vi "_PC_RTFunc_AccessLaser.vi"(7 "Function":enum16{"Init", "Write", "Read"}(ring), 8 "error in (no error)":errorcluster, 10 "Data":variant) -> (0 "error out":errorcluster, 2 "LaserSetting":T1={"Energy"=1.0, "Freq"=1.0, "Emission"=FALSE, "TriggerSource"=enum."Internal", "Time Stamp"=timestamp(0 s since 1904-01-01)})   [LabVIEW 2018]
uses:
  RT/ControlLoop/Laser/Ctl/_ctl_LaserParam.ctl
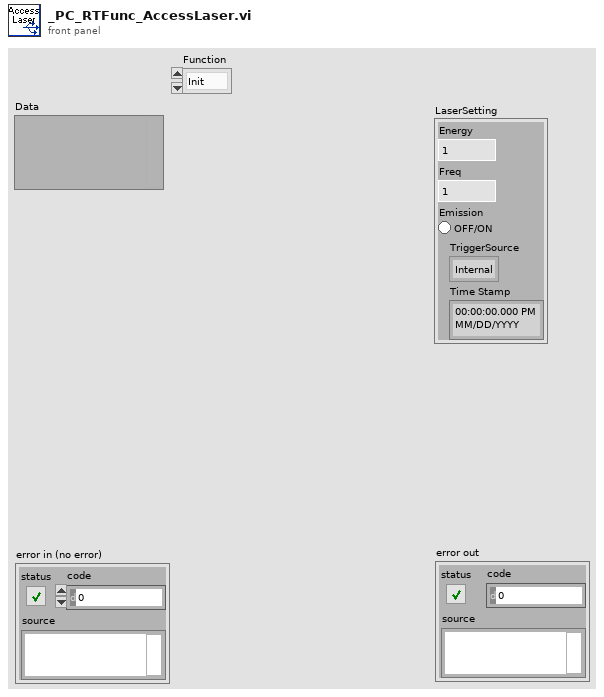
[diagram p1: front panel]
types:
  T1 = typedef "_ctl_LaserParam.ctl" = cluster{"Energy":dbl, "Freq":dbl, "Emission":bool, "TriggerSource":enum16{"Internal", "External"}, "Time Stamp":timestamp}
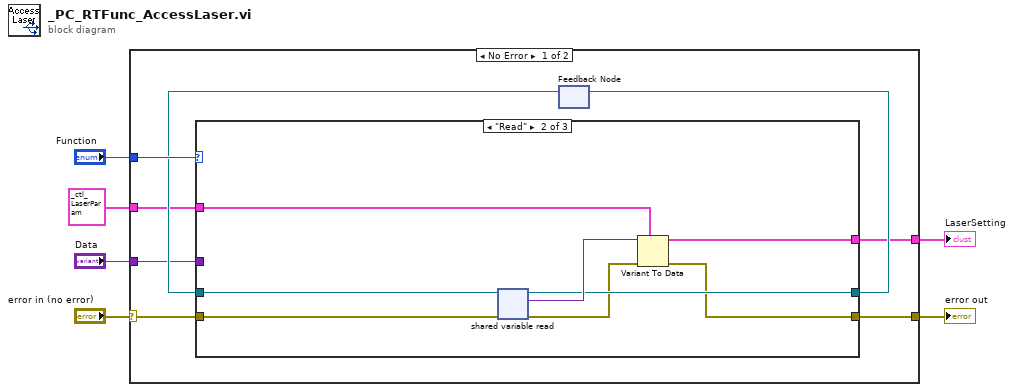
[diagram p0: block diagram]
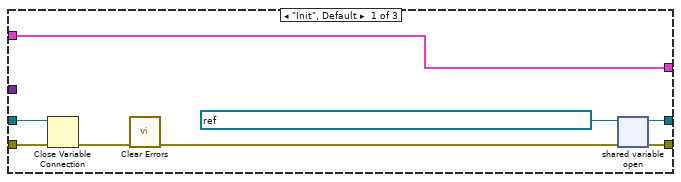
[diagram p2: hidden frame]
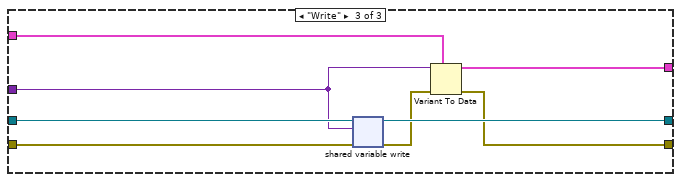
[diagram p3: hidden frame]
diagram:
  n1 = case shown="No Error" "error in (no error)" {
    selector: "error in (no error)" -> [w11 w39]
    tunnel: "Function" -> [w14 _]
    tunnel: [w10 w39] -> w4
    tunnel: T1 {"Energy"=50.0, "Freq"=100.0, "Emission"=FALSE, "TriggerSource"=enum."Internal", "Time Stamp"=timestamp(0 s since 1904-01-01)} ("LaserSetting") -> [w9 w40]
    tunnel: [w8 w40] -> w2
    tunnel: "Data" -> [w7 _]
    frame No Error {
      n2 = feedback #1() -> (w12:refnum<k21>)  [unwired: 1 in]
      n3 = case shown="\"Read\"" w14 {
        tunnel: w12 -> [w18 w30 w38]
        tunnel: [w21 w26 w36] -> w13
        tunnel: w11 -> [w17 w29 w37]
        tunnel: [w20 w24 w31] -> w10
        tunnel: w9 -> [w19 w28 w34]
        tunnel: [w19 w23 w33] -> w8
        tunnel: w7 -> [_ _ w35]
        frame "Init", Default {
          n4 = Close Variable Connection(8:w17, 11:w18) -> (0:w16:errorcluster)
          n5 = call <vilib>:"Clear Errors.vi"("error in (no error)"=w16) -> ("error out"=w15:errorcluster)  [unwired: 5 in, 1 out]
          n6 = shared-variable-open(refnum<k21> "ni.var.psp://NI-sbRIO/_RT_CtrlLoop_Laser_Variables/LaserSetting" ("shared variable refnum in"), w15) -> (w21:refnum<k21>, w20:errorcluster)
        }
        frame "Read" {
          n7 = shared-variable-read(w30, w29) -> (w26:refnum<k21>, w25:errorcluster, w27:variant)
          n8 = Variant To Data(error in=w25, type=w28, Variant=w27) -> (data=w23:T1, error out=w24:errorcluster)
        }
        frame "Write" {
          n9 = shared-variable-write(w38, w37, w35) -> (w36:refnum<k21>, w32:errorcluster)
          n10 = Variant To Data(error in=w32, type=w34, Variant=w35) -> (data=w33:T1, error out=w31:errorcluster)
        }
      }
      n11 = feedback-in #1(w13) -> ()
    }
    frame Error {
    }
  }
  "error out" <- w4
  "LaserSetting" <- w2
